vi "elimination.vi"(3 "index to compare":u8, 5 "input equations":T1[](array[typedef])) -> (1 "x-y":T1)   [LabVIEW 2009]
uses:
  polynomial equation.ctl
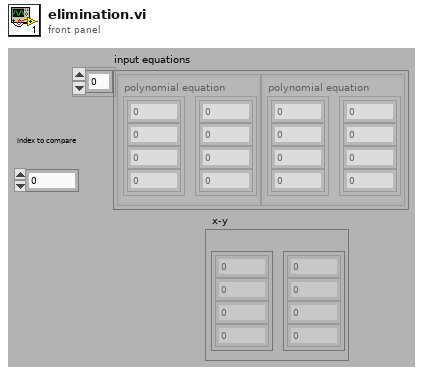
[diagram p1: front panel]
types:
  T1 = typedef "polynomial equation.ctl" = cluster{"i":dbl[], "ii":dbl[]}
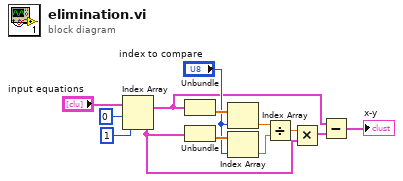
[diagram p0: block diagram]
diagram:
  n1 = Index Array(array="input equations", index #1=0, index #2=1) -> (element #1=w2:T1, element #2=w4:T1)
  n2 = Unbundle(w2) -> ("ii"=w9:dbl[])  [unwired: 1 out]
  n3 = Unbundle(w4) -> ("ii"=w10:dbl[])  [unwired: 1 out]
  n4 = Index Array(array=w9, index="index to compare") -> (element=w7:dbl)
  n5 = Index Array(array=w10, index="index to compare") -> (element=w6:dbl)
  n6 = Divide(x=w7, y=w6) -> (x/y=w5:dbl)
  n7 = Multiply(x=w5, y=w4) -> (x*y=w3:T1)
  n8 = Subtract(x=w2, y=w3) -> (x-y=→"x-y":T1)
